vi "Data to XY Plot.vi"(0 "VISA resource name":refnum<visa-resource-name>, 1 "Zero Time Axis (T)":bool=TRUE, 7 "String of Data":string) -> (8 "XY Graph":cluster{dbl[], dbl[]}(graph))   [LabVIEW 2024, in "Keithley 648X Series.lvlib"]
doc: "This private VI converts a string of data to an XY Plot. The method used to convert said string differs based on the VISA connection type."
uses:
  <instrlib>/Keithley 648X Series/Keithley 648X Series.lvlib
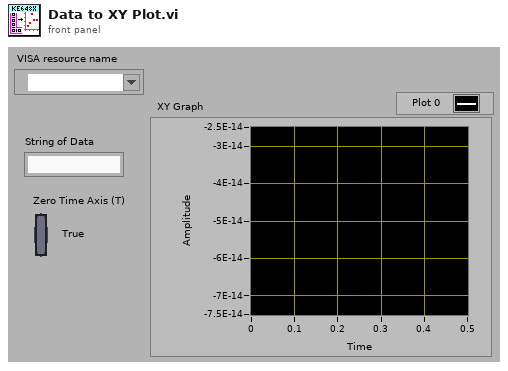
[diagram p1: front panel]
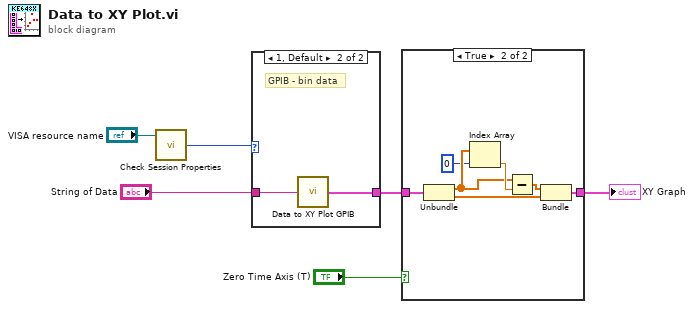
[diagram p0: block diagram]
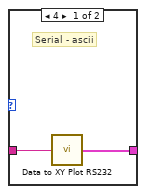
[diagram p3: hidden frame]
diagram:
  n1 = call <instrlib>:"Check Session Properties.vi"("VISA resource name"="VISA resource name") -> ("Interface Type"=w4:u16)  [unwired: 11 in, 3 out]
  n2 = case shown="1, Default" w4 {
    tunnel: "String of Data" -> [w8 w10]
    tunnel: [w7 w9] -> w2
    frame 4 {
      # "Serial - ascii"
      n3 = call <instrlib>:"Data to XY Plot RS232.vi"("Input String"=w8) -> ("XY Graph"=w7:cluster{dbl[], dbl[]})  [unwired: 14 in]
    }
    frame 1, Default {
      # "GPIB - bin data"
      n4 = call <instrlib>:"Data to XY Plot GPIB.vi"("String of Data"=w10) -> ("XY Graph"=w9:cluster{sgl[], sgl[]})  [unwired: 14 in]
    }
  }
  n5 = case shown="True" "Zero Time Axis (T)" {
    tunnel: w2 -> [w11 w18]
    tunnel: [w11 w13] -> w1
    frame False {
    }
    frame True {
      n6 = Unbundle(w18) -> (w16:dbl[], w14:dbl[])
      n7 = Index Array(array=w16, index=0) -> (element=w17:dbl)
      n8 = Subtract(x=w16, y=w17) -> (x-y=w15:dbl[])
      n9 = Bundle(w15, w14) -> (w13:cluster{dbl[], dbl[]})  [unwired: 1 in]
    }
  }
  "XY Graph" <- w1
